vi "Excel Sort Data.vi"(0 "report in":refnum<class "NI_report.lvclass">, 1 "order (ascend)":i32(ring)=1 items=["xlAscending"=1, "xlDescending"=2], 5 "from (0, 0)":cluster{"row":i32, "column":i32}, 7 "start (0, 0)":cluster{"row":i32, "column":i32}, 9 "end (0, 0)":cluster{"row":i32, "column":i32}, 11 "error in (no error)":errorcluster, 12 "orientation (rows)":i32(ring)=2 items=["xlSortRows"=2, "xlSortColumns"=1]) -> (4 "report out":refnum<class "NI_report.lvclass">, 15 "error out":errorcluster)   [LabVIEW 2017, in "NI_Excel.lvclass"]
doc: "Sorts the range of cells specified by the <B>start</B> and <B>end</B> clusters."
uses:
  <vilib>/Utility/NIReport.llb/Excel/NI_Excel.lvclass
  <vilib>/Utility/NIReport.llb/NI_report.lvclass
  C:/Program Files (x86)/National Instruments/LabVIEW 2017/vi.lib/Utility/NIReport.llb/NI_report.lvclass
  <vilib>/Utility/NIReport.llb/Excel/NI_Excel.lvclass/NI_Excel.ctl
  <vilib>/Utility/NIReport.llb/NI_ReportGenerationCore.lvlib
  <vilib>/addons/_office/NI_ReportGenerationToolkit.lvlib
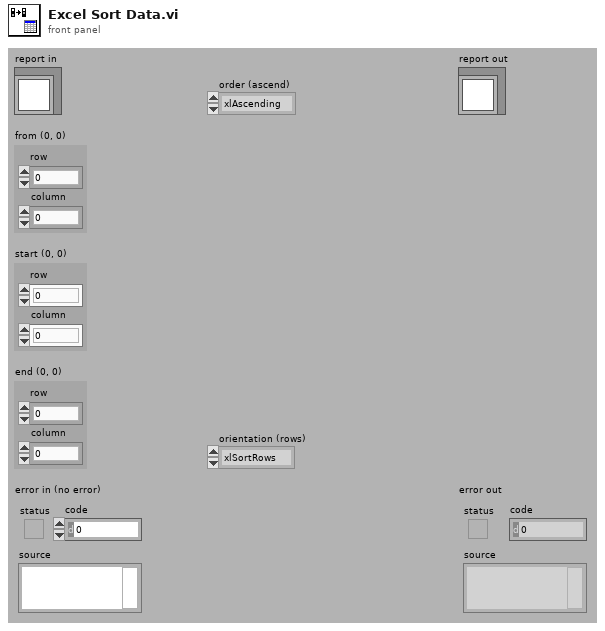
[diagram p1: front panel]
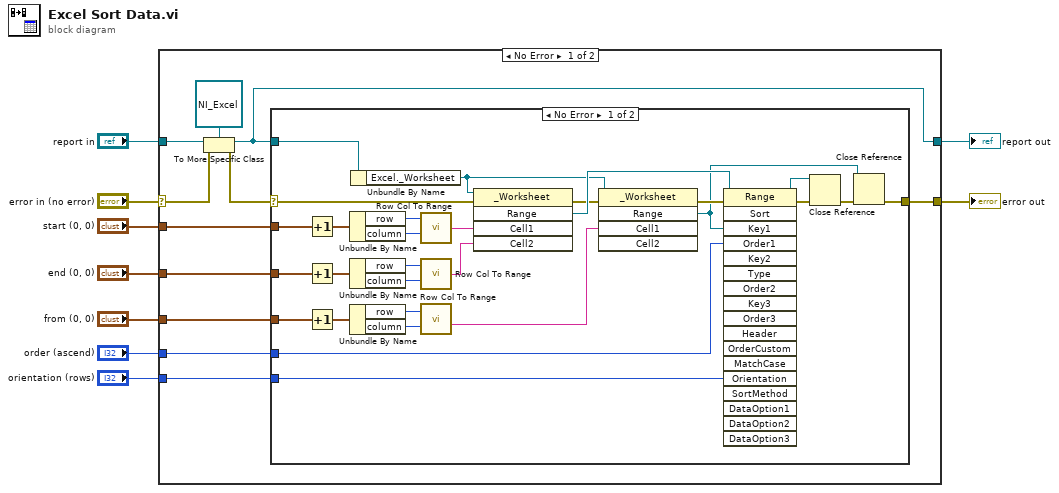
[diagram p0: block diagram]
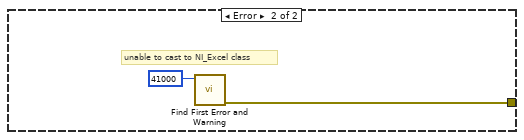
[diagram p2: hidden frame]
diagram:
  n1 = case shown="No Error" "error in (no error)" {
    selector: "error in (no error)" -> [w10 w52]
    tunnel: [w15 w52] -> w8
    tunnel: [w12 w51] -> w6
    tunnel: "report in" -> [w13 w51]
    tunnel: "start (0, 0)" -> [w20 _]
    tunnel: "end (0, 0)" -> [w19 _]
    tunnel: "from (0, 0)" -> [w18 _]
    tunnel: "order (ascend)" -> [w17 _]
    tunnel: "orientation (rows)" -> [w16 _]
    frame No Error {
      n2 = To More Specific Class(target class=refnum<class "NI_Excel.lvclass"> refnum ("report in"), reference=w13, error in=w10) -> (specific class reference=w12:refnum<class "NI_Excel.lvclass">, error out=w11:errorcluster)
      n3 = case shown="No Error" w11 {
        selector: w11 -> [w21 _]
        tunnel: w20 -> [w32 _]
        tunnel: w19 -> [w31 _]
        tunnel: w18 -> [w30 _]
        tunnel: w17 -> [w29 _]
        tunnel: w16 -> [w28 _]
        tunnel: [w25 w49] -> w15
        tunnel: w12 -> [w22 _]
        frame No Error {
          n4 = Increment(x=w32) -> (x+1=w45:cluster{"row":i32, "column":i32})
          n5 = Increment(x=w31) -> (x+1=w46:cluster{"row":i32, "column":i32})
          n6 = Increment(x=w30) -> (x+1=w47:cluster{"row":i32, "column":i32})
          n7 = Unbundle By Name(w45) -> ("row"=w39:i32, "column"=w40:i32)
          n8 = Unbundle By Name(w46) -> ("row"=w41:i32, "column"=w42:i32)
          n9 = Unbundle By Name(w47) -> ("row"=w43:i32, "column"=w44:i32)
          n10 = Unbundle By Name(w22) -> ("Excel._Worksheet"=w24:refnum<k7>)
          n11 = call <vilib>:"Row Col To Range.vi"("Column"=w40, "Row"=w39) -> ("Output String"=w38:string)
          n12 = call <vilib>:"Row Col To Range.vi"("Column"=w42, "Row"=w41) -> ("Output String"=w37:string)
          n13 = call <vilib>:"Row Col To Range.vi"("Column"=w44, "Row"=w43) -> ("Output String"=w33:string)
          n14 = invoke class="_Worksheet" method="Range"(reference=w24, error in=w21, "Cell1"=w38, "Cell2"=w37) -> (error out=w27:errorcluster, "Range"=w36:refnum<k7>)  [unwired: 1 in, 3 out]
          n15 = invoke class="_Worksheet" method="Range"(reference=w24, error in=w27, "Cell1"=w33) -> (error out=w26:errorcluster, "Range"=w23:refnum<k7>)  [unwired: 2 in, 3 out]
          n16 = invoke class="Range" method="Sort"(reference=w36, error in=w26, "Key1"=w23, "Order1"=w29, "Orientation"=w28) -> (reference out=w34:refnum<k7>, error out=w35:errorcluster)  [unwired: 13 in, 16 out]
          n17 = Close Reference(reference=w34, error in (no error)=w35) -> (error out=w48:errorcluster)
          n18 = Close Reference(reference=w23, error in (no error)=w48) -> (error out=w25:errorcluster)
        }
        frame Error {
          # "unable to cast to NI_Excel class"
          n19 = call <vilib>:"Find First Error and Warning.vi"("error code"=41000) -> ("error out"=w49:errorcluster)  [unwired: 2 in, 4 out]
        }
      }
    }
    frame Error {
    }
  }
  "error out" <- w8
  "report out" <- w6
